vi "Start CANFD Session.vi"(11 "CAN Interface":refnum<k21>="CAN1") -> (0 "Tester Write Session out":refnum<k21>, 1 "Read Session out":refnum<k21>, 3 "DSC Write Session out":refnum<k21>)   [LabVIEW 2018]
uses:
  <vilib>/xnet/xnet.llb/XNET CAN Comm State.ctl
  <vilib>/xnet/xnet.llb/XNET Control Scope.ctl
  <vilib>/xnet/xnet.llb/XNET Frame CAN.ctl
  <vilib>/xnet/xnet.llb/XNET Frame Type CAN.ctl
  <vilib>/xnet/xnet.llb/XNET Create Session (Frame Input Queued).vi
  <vilib>/xnet/xnet.llb/XNET Create Session (Frame Output Single-point).vi
  <vilib>/xnet/xnet.llb/XNET Write (Frame CAN).vi
  <vilib>/xnet/xnet.llb/XNET Read (State CAN Comm).vi
  <vilib>/xnet/xnet.llb/XNET Wait (Interface Communicating).vi
  <resource>/objmgr/xnet.rc
panel:
  in  "error in (no error)":errorcluster
  out "TesterPresentSession":refnum<k21>
  out "CAN:I/O Mode":u32(ring) items=["CAN 2.0", "CAN FD", "CAN FD+BRS"]
  out "Protocol":u32(ring) items=["CAN", "FlexRay", "LIN"]
  out "CAN:Transceiver Capability":u32(ring) items=["HS"=0, "LS"=1, "XS"=3, "XS (HS/LS)"=4]
  out "Interface:CAN:Transceiver State":u32(ring) items=["Normal", "Sleep", "Single Wire Wakeup", "Single Wire High-Speed"]
  out "Interface:CAN:Transceiver State 2":u32(ring) items=["Normal", "Sleep", "Single Wire Wakeup", "Single Wire High-Speed"]
  out "Interface:CAN:Transceiver State 3":u32(ring) items=["Normal", "Sleep", "Single Wire Wakeup", "Single Wire High-Speed"]
  out "CAN:Termination Capability":u32(ring) items=["No", "Yes"]
  out "Array":T1[](array[typedef]) items=["Error Active", "Error Passive", "Bus Off", "Init"]
  out "error out":errorcluster
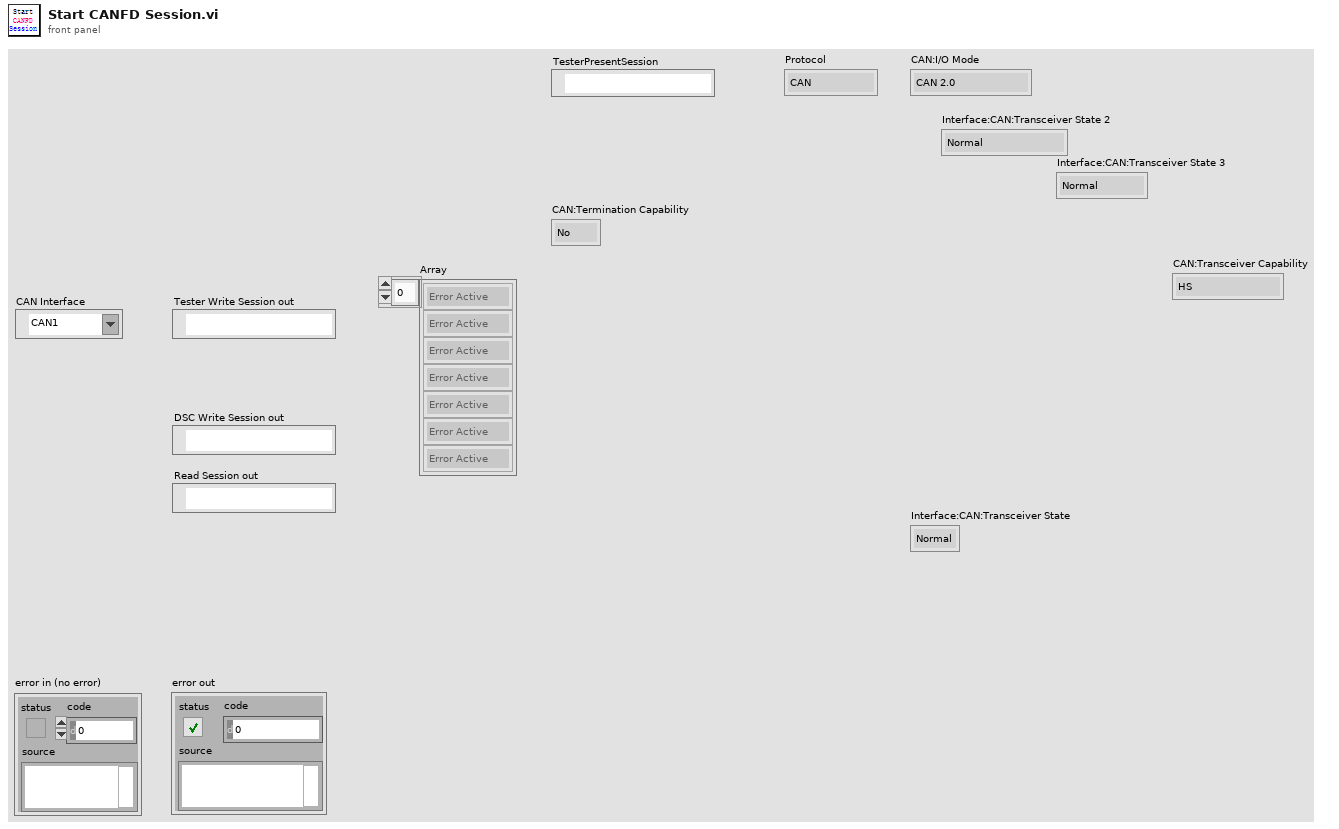
[diagram p1: front panel]
types:
  T1 = typedef "XNET CAN Comm State.ctl" = u8
  T2 = typedef "XNET Frame CAN.ctl" = cluster{"timestamp":timestamp, "payload":u8[], "identifier":u32, "type":T3, "extended?":bool, "echo?":bool}
  T3 = typedef "XNET Frame Type CAN.ctl" = u8
  T4 = typedef "XNET Control Scope.ctl" = u32
  T5 = cluster{"Comment":string, "Default Payload":u8[], "Identifier":u32, "Name (Short)":string, "Payload Length":u32, "PDU_Mapping":cluster{"PDU":string, "Start Bit":u32, "Update Bit":i32}[], "CAN:Extended Identifier?":bool, "CAN:Timing Type":u32, "CAN:Transmit Time":dbl, "CAN:I/O Mode":u32}
  T6 = typedef "XNET CAN Comm.ctl" = cluster{"fault code":i32, "fault?":bool, "communication state":T1, "last error":T7, "receive error counter":u8, "transmit error counter":u8, "transceiver error?":bool, "sleep?":bool}
  T7 = typedef "XNET CAN Last Err.ctl" = u8
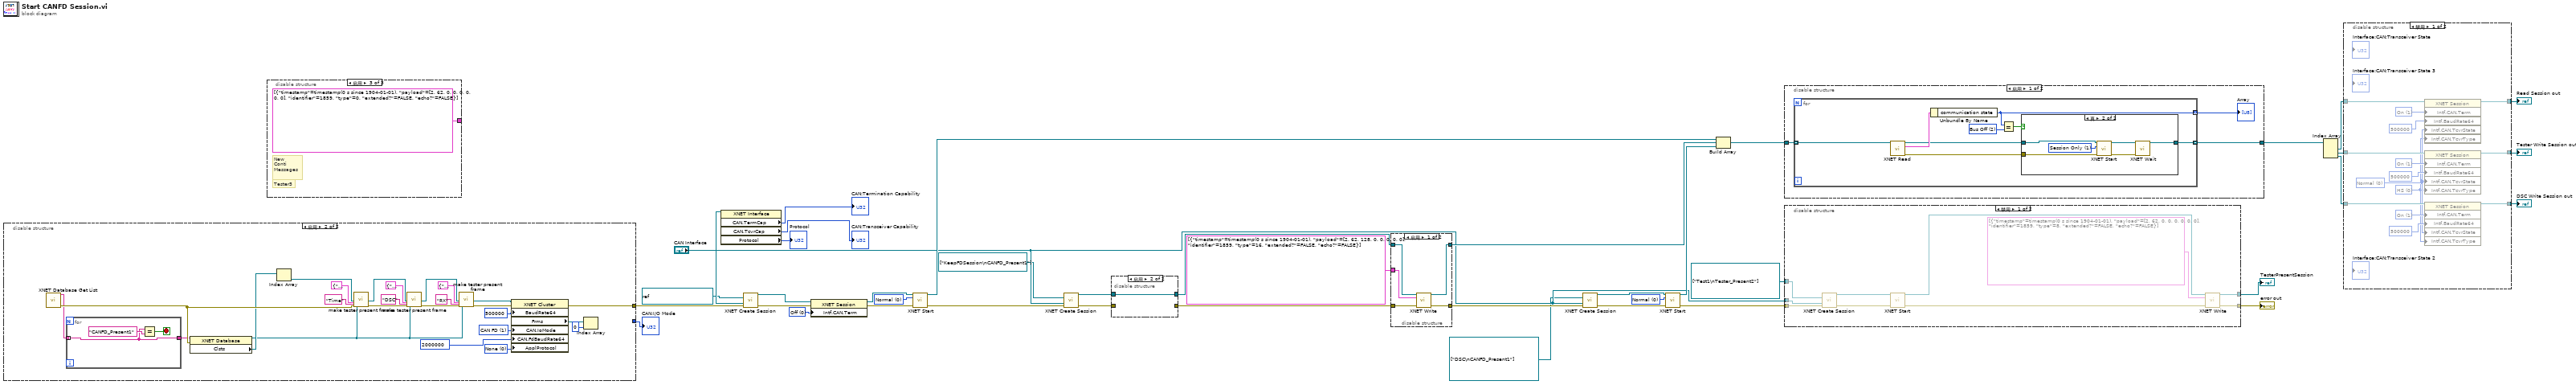
[diagram p0: block diagram]
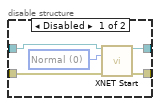
[diagram p3: hidden frame]
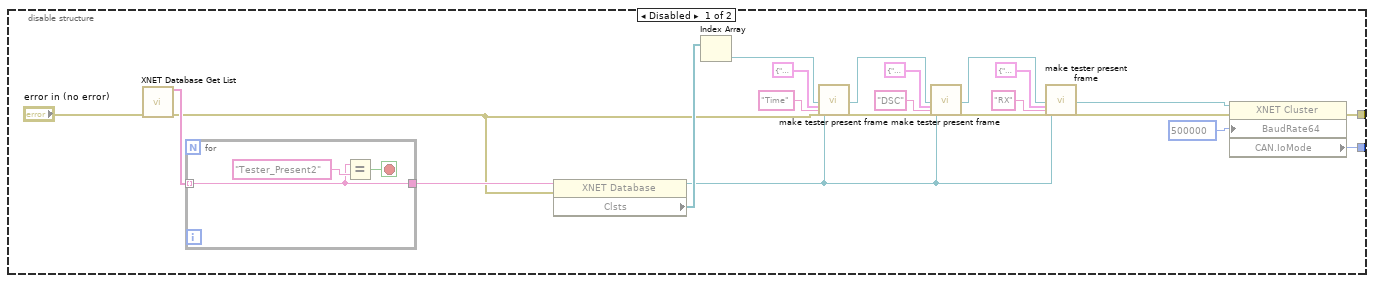
[diagram p4: hidden frame]
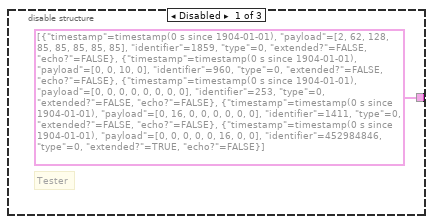
[diagram p9: hidden frame]
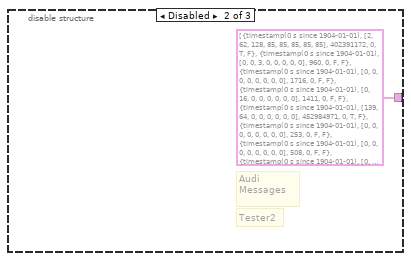
[diagram p10: hidden frame]
diagram:
  w11 = u32 0 items=["Off", "On"] ("Interface:CAN:Termination")
  w29 = T4 0 items=["Normal", "Session Only", "Interface Only", "Session Only Blocking"] ("scope (normal)")
  w30 = T4 0 items=["Normal", "Session Only", "Interface Only", "Session Only Blocking"] ("scope (normal)")
  n1 = disable-structure shown="启用" {
    disable-tunnel: [w60 w69] -> w40
    disable-tunnel: [w41 _] -> w15
    frame Disabled {
      n2 = call <vilib>:"XNET Database Get List.vi"("error in (no error)"="error in (no error)") -> ("array of alias"=w50:string[], "error out"=w46:errorcluster)  [unwired: 12 in, 1 out]
      n3 = for {
        tunnel: w50 -> [w63] mode=indexing
        tunnel: [w63] -> w49
        stop <- w64 stop-if-true
        n4 = Equal?(x=w63, y="Tester_Present2") -> (x = y?=w64:bool)
      }
      n5 = property class="XNET Database"(reference=w49, error in=w46) -> (reference out=w42:refnum<k21>, "Clsts"=w61:refnum<k21>[])  [unwired: 1 out]
      n6 = Index Array(array=w61) -> (element=w44:refnum<k21>)  [unwired: 1 in]
      n7 = call "make tester present frame.vi"("Cluster::"=w44, "New Frame Properties"=T5 {"Comment"="DSC", "Default Payload"=[0, 0, 0, 0, 0, 0, 0, 0], "Identifier"=1714, "Name (Short)"="Time", "Payload Length"=8, "PDU_Mapping"=[], "CAN:Extended Identifier?"=FALSE, "CAN:Timing Type"=0, "CAN:Transmit Time"=0.001, "CAN:I/O Mode"=0}, "frame name"="Time", "error in (no error)"=w46, "database in"=w42) -> ("target cluster out"=w43:refnum<k21>, "error out"=w45:errorcluster)  [unwired: 21 in]
      n8 = call "make tester present frame.vi"("Cluster::"=w43, "New Frame Properties"=T5 {"Comment"="DSC", "Default Payload"=[0, 0, 0, 0, 0, 0, 0, 0], "Identifier"=402391172, "Name (Short)"="DSC", "Payload Length"=8, "PDU_Mapping"=[], "CAN:Extended Identifier?"=TRUE, "CAN:Timing Type"=1, "CAN:Transmit Time"=0.001, "CAN:I/O Mode"=0}, "frame name"="DSC", "error in (no error)"=w45, "database in"=w42) -> ("target cluster out"=w59:refnum<k21>, "error out"=w58:errorcluster)  [unwired: 21 in]
      n9 = call "make tester present frame.vi"("Cluster::"=w59, "New Frame Properties"=T5 {"Comment"="RX", "Default Payload"=[0, 127, 0, 0, 0, 0, 0, 0], "Identifier"=402522244, "Name (Short)"="RX", "Payload Length"=8, "PDU_Mapping"=[], "CAN:Extended Identifier?"=TRUE, "CAN:Timing Type"=1, "CAN:Transmit Time"=0.001, "CAN:I/O Mode"=0}, "frame name"="RX", "error in (no error)"=w58, "database in"=w42) -> ("target cluster out"=w52:refnum<k21>, "error out"=w51:errorcluster)  [unwired: 21 in]
      n10 = property class="XNET Cluster"(reference=w52, error in=w51, "BaudRate64"=u64 500000 ("64bit Baud Rate")) -> (error out=w60:errorcluster, "CAN.IoMode"=w41:u32)  [unwired: 1 out]
    }
    frame Enabled {
      w67 = u32 0 items=["None", "J1939"] ("Application Protocol")
      w68 = u32 1 items=["CAN 2.0", "CAN FD", "CAN FD+BRS"] ("CAN:I/O Mode")
      n11 = call <vilib>:"XNET Database Get List.vi"() -> ("array of alias"=w87:string[], "error out"=w88:errorcluster)  [unwired: 13 in, 1 out]
      n12 = for {
        tunnel: w87 -> [w91] mode=indexing
        tunnel: [w91] -> w74
        stop <- w92 stop-if-true
        n13 = Equal?(x=w91, y="CANFD_Present1") -> (x = y?=w92:bool)
      }
      n14 = property class="XNET Database"(reference=w74, error in=w88) -> (reference out=w71:refnum<k21>, "Clsts"=w75:refnum<k21>[])  [unwired: 1 out]
      n15 = Index Array(array=w75) -> (element=w90:refnum<k21>)  [unwired: 1 in]
      n16 = call "make tester present frame.vi"("Cluster::"=w90, "New Frame Properties"=T5 {"Comment"="Time", "Default Payload"=[0, 0, 0, 0, 0, 0, 0, 0], "Identifier"=1859, "Name (Short)"="Time", "Payload Length"=8, "PDU_Mapping"=[], "CAN:Extended Identifier?"=FALSE, "CAN:Timing Type"=0, "CAN:Transmit Time"=0.1, "CAN:I/O Mode"=0}, "frame name"="Time", "error in (no error)"=w88, "database in"=w71) -> ("target cluster out"=w70:refnum<k21>, "error out"=w89:errorcluster)  [unwired: 21 in]
      n17 = call "make tester present frame.vi"("Cluster::"=w70, "New Frame Properties"=T5 {"Comment"="DSC", "Default Payload"=[0, 0, 0, 16, 1, 0, 0, 0], "Identifier"=1859, "Name (Short)"="DSC", "Payload Length"=8, "PDU_Mapping"=[], "CAN:Extended Identifier?"=FALSE, "CAN:Timing Type"=1, "CAN:Transmit Time"=0.0, "CAN:I/O Mode"=0}, "frame name"="DSC", "error in (no error)"=w89, "database in"=w71) -> ("target cluster out"=w83:refnum<k21>, "error out"=w84:errorcluster)  [unwired: 21 in]
      n18 = call "make tester present frame.vi"("Cluster::"=w83, "New Frame Properties"=T5 {"Comment"="RX", "Default Payload"=[0, 127, 0, 0, 0, 0, 0, 0], "Identifier"=1867, "Name (Short)"="RX", "Payload Length"=8, "PDU_Mapping"=[], "CAN:Extended Identifier?"=FALSE, "CAN:Timing Type"=1, "CAN:Transmit Time"=0.0, "CAN:I/O Mode"=1}, "frame name"="RX", "error in (no error)"=w84, "database in"=w71) -> ("target cluster out"=w85:refnum<k21>, "error out"=w86:errorcluster)  [unwired: 21 in]
      n19 = property class="XNET Cluster"(reference=w85, error in=w86, "BaudRate64"=u64 500000 ("64bit Baud Rate"), "CAN.IoMode"=w68, "CAN.FdBaudRate64"=u64 2000000 ("CAN:64bit FD Baud Rate"), "ApplProtocol"=w67) -> (error out=w69:errorcluster, "Frms"=w73:refnum<k21>[])  [unwired: 1 out]
      n20 = Index Array(array=w73, index=0 ("索引")) -> ()  [unwired: 1 out]
    }
  }
  "CAN:I/O Mode" <- w15
  n21 = disable-structure shown="启用" {
    disable-tunnel: [T2[] [{"timestamp"=timestamp(0 s since 1904-01-01), "payload"=[2, 62, 128, 85, 85, 85, 85, 85], "identifier"=1859, "type"=0, "extended?"=FALSE, "echo?"=FALSE}, {"timestamp"=timestamp(0 s since 1904-01-01), "payload"=[0, 0, 10, 0], "identifier"=960, "type"=0, "extended?"=FALSE, "echo?"=FALSE}, {"timestamp"=timestamp(0 s since 1904-01-01), "payload"=[0, 0, 0, 0, 0, 0, 0, 0], "identifier"=253, "type"=0, "extended?"=FALSE, "echo?"=FALSE}, {"timestamp"=timestamp(0 s since 1904-01-01), "payload"=[0, 16, 0, 0, 0, 0, 0, 0], "identifier"=1411, "type"=0, "extended?"=FALSE, "echo?"=FALSE}, {"timestamp"=timestamp(0 s since 1904-01-01), "payload"=[0, 0, 0, 0, 0, 16, 0, 0], "identifier"=452984846, "type"=0, "extended?"=TRUE, "echo?"=FALSE}] ("data") T2[] [{"timestamp"=timestamp(0 s since 1904-01-01), "payload"=[2, 62, 128, 85, 85, 85, 85, 85], "identifier"=402391172, "type"=0, "extended?"=TRUE, "echo?"=FALSE}, {"timestamp"=timestamp(0 s since 1904-01-01), "payload"=[0, 0, 3, 0, 0, 0, 0, 0], "identifier"=960, "type"=0, "extended?"=FALSE, "echo?"=FALSE}, {"timestamp"=timestamp(0 s since 1904-01-01), "payload"=[0, 0, 0, 0, 0, 0, 0, 0], "identifier"=1716, "type"=0, "extended?"=FALSE, "echo?"=FALSE}, {"timestamp"=timestamp(0 s since 1904-01-01), "payload"=[0, 16, 0, 0, 0, 0, 0, 0], "identifier"=1411, "type"=0, "extended?"=FALSE, "echo?"=FALSE}, {"timestamp"=timestamp(0 s since 1904-01-01), "payload"=[139, 64, 0, 0, 0, 0, 0, 0], "identifier"=452984971, "type"=0, "extended?"=TRUE, "echo?"=FALSE}, {"timestamp"=timestamp(0 s since 1904-01-01), "payload"=[0, 0, 0, 0, 0, 0, 0, 0], "identifier"=253, "type"=0, "extended?"=FALSE, "echo?"=FALSE}, {"timestamp"=timestamp(0 s since 1904-01-01), "payload"=[0, 0, 0, 0, 0, 0, 0, 0], "identifier"=508, "type"=0, "extended?"=FALSE, "echo?"=FALSE}, {"timestamp"=timestamp(0 s since 1904-01-01), "payload"=[0, 0, 0, 0, 150, 0, 0, 0], "identifier"=1646, "type"=0, "extended?"=FALSE, "echo?"=FALSE}, {"timestamp"=timestamp(0 s since 1904-01-01), "payload"=[0, 0, 0, 0, 0, 0, 0, 150], "identifier"=1719, "type"=0, "extended?"=FALSE, "echo?"=FALSE}, {"timestamp"=timestamp(0 s since 1904-01-01), "payload"=[0, 0, 4, 0, 0, 0, 0, 0], "identifier"=958, "type"=0, "extended?"=FALSE, "echo?"=FALSE}, {"timestamp"=timestamp(0 s since 1904-01-01), "payload"=[0, 0, 0, 0, 0, 0, 0, 0], "identifier"=1635, "type"=0, "extended?"=FALSE, "echo?"=FALSE}, {"timestamp"=timestamp(0 s since 1904-01-01), "payload"=[0, 0, 0, 0, 0, 0, 0, 0], "identifier"=319, "type"=0, "extended?"=FALSE, "echo?"=FALSE}, {"timestamp"=timestamp(0 s since 1904-01-01), "payload"=[0, 0, 0, 0, 0, 0, 0, 0], "identifier"=1616, "type"=0, "extended?"=FALSE, "echo?"=FALSE}, {"timestamp"=timestamp(0 s since 1904-01-01), "payload"=[0, 12, 0, 0, 0, 0, 0, 0], "identifier"=1413, "type"=0, "extended?"=FALSE, "echo?"=FALSE}, {"timestamp"=timestamp(0 s since 1904-01-01), "payload"=[0, 0, 0, 0, 0, 0, 0, 0], "identifier"=1462, "type"=0, "extended?"=FALSE, "echo?"=FALSE}, {"timestamp"=timestamp(0 s since 1904-01-01), "payload"=[16, 64, 0, 0, 0, 16, 0, 0], "identifier"=452984848, "type"=0, "extended?"=TRUE, "echo?"=FALSE}, {"timestamp"=timestamp(0 s since 1904-01-01), "payload"=[0, 0, 0, 0, 0, 0, 0, 0], "identifier"=976, "type"=0, "extended?"=FALSE, "echo?"=FALSE}, {"timestamp"=timestamp(0 s since 1904-01-01), "payload"=[0, 0, 0, 0, 0, 0, 0, 0], "identifier"=974, "type"=0, "extended?"=FALSE, "echo?"=FALSE}, {"timestamp"=timestamp(0 s since 1904-01-01), "payload"=[74, 64, 0, 0, 0, 0, 0, 0], "identifier"=452984906, "type"=0, "extended?"=TRUE, "echo?"=FALSE}, {"timestamp"=timestamp(0 s since 1904-01-01), "payload"=[0, 0, 0, 0, 0, 0, 0, 0], "identifier"=977, "type"=0, "extended?"=FALSE, "echo?"=FALSE}, {"timestamp"=timestamp(0 s since 1904-01-01), "payload"=[0, 0, 0, 0, 0, 0, 0, 0], "identifier"=975, "type"=0, "extended?"=FALSE, "echo?"=FALSE}, {"timestamp"=timestamp(0 s since 1904-01-01), "payload"=[75, 64, 0, 0, 0, 0, 0, 0], "identifier"=452984907, "type"=0, "extended?"=TRUE, "echo?"=FALSE}] ("Array 3") T2[] [{"timestamp"=timestamp(0 s since 1904-01-01), "payload"=[2, 62, 0, 0, 0, 0, 0, 0], "identifier"=1859, "type"=0, "extended?"=FALSE, "echo?"=FALSE}] ("data")] -> _
    frame Disabled {
      # "Tester"
    }
    frame Disabled {
      # "Tester2"
      # "Audi\nMessages"
    }
    frame Enabled {
      # "Tester3"
      # "New\nConti\nMessages"
    }
  }
  n22 = property class="XNET Interface"(reference="CAN Interface") -> ("CAN.TermCap"=→"CAN:Termination Capability":u32, "CAN.TcvrCap"=→"CAN:Transceiver Capability":u32, "Protocol"=→"Protocol":u32)  [unwired: 1 in, 2 out]
  n23 = call-poly <vilib>:"XNET Create Session.vi"("frame"=refnum<k21> "RX\nCANFD_Present1" ("XNET Frame"), "interface"="CAN Interface", "error in (no error)"=w40) -> ("session out"=w14:refnum<k21>, "error out"=w12:errorcluster)  [unwired: 11 in]
  n24 = property class="XNET Session"(reference=w14, error in=w12, "Intf.CAN.Term"=w11) -> (reference out=w13:refnum<k21>, error out=w10:errorcluster)
  n25 = call <vilib>:"XNET Start.vi"("session in"=w13, "scope (normal)"=w30, "error in (no error)"=w10) -> ("session out"=w37:refnum<k21>, "error out"=w32:errorcluster)  [unwired: 11 in]
  n26 = call-poly <vilib>:"XNET Create Session.vi"("frame list"=refnum<k21>[] ["KeepFDSession\nCANFD_Present1"] ("Frames"), "interface"="CAN Interface", "error in (no error)"=w32) -> ("session out"=w27:refnum<k21>, "error out"=w28:errorcluster)  [unwired: 11 in]
  n27 = disable-structure shown="启用" {
    disable-tunnel: [w101 w102] -> w39
    disable-tunnel: [w100 _] -> w38
    disable-tunnel: w28 -> [w98 _]
    disable-tunnel: w27 -> [w97 w102]
    frame Disabled {
      w99 = T4 0 items=["Normal", "Session Only", "Interface Only", "Session Only Blocking"] ("scope (normal)")
      n28 = call <vilib>:"XNET Start.vi"("session in"=w97, "scope (normal)"=w99, "error in (no error)"=w98) -> ("session out"=w101:refnum<k21>, "error out"=w100:errorcluster)  [unwired: 11 in]
    }
    frame Enabled {
    }
  }
  n29 = disable-structure shown="启用" {
    disable-tunnel: w39 -> [w107 w108]
    disable-tunnel: w38 -> [w106 w109]
    disable-tunnel: [w105 w108] -> w36
    disable-tunnel: [w104 w109] -> w31
    disable-tunnel: T2[] [{"timestamp"=timestamp(0 s since 1904-01-01), "payload"=[2, 62, 128, 0, 0, 0, 0, 0], "identifier"=1859, "type"=16, "extended?"=FALSE, "echo?"=FALSE}] ("data") -> [w103 _]
    frame Enabled {
      n30 = call-poly <vilib>:"XNET Write.vi"("session in"=w107, "data"=w103, "error in (no error)"=w106) -> ("session out"=w105:refnum<k21>, "error out"=w104:errorcluster)  [unwired: 11 in]
    }
    frame Disabled {
    }
  }
  n31 = call-poly <vilib>:"XNET Create Session.vi"("frame list"=refnum<k21>[] ["DSC\nCANFD_Present1"] ("Frames"), "interface"="CAN Interface", "error in (no error)"=w31) -> ("session out"=w26:refnum<k21>, "error out"=w25:errorcluster)  [unwired: 11 in]
  n32 = call <vilib>:"XNET Start.vi"("session in"=w26, "scope (normal)"=w29, "error in (no error)"=w25) -> ("session out"=w35:refnum<k21>, "error out"=w6:errorcluster)  [unwired: 11 in]
  n33 = Build Array(w37, w36, w35) -> (w34:refnum<k21>[])
  n34 = disable-structure shown="启用" {
    disable-tunnel: w34 -> [w112 w128]
    disable-tunnel: [w110 w128] -> w33
    frame Enabled {
      n35 = for {
        tunnel: w112 -> [w119] mode=indexing
        tunnel: [w114] -> w111 mode=indexing
        tunnel: [w113] -> w110 mode=indexing
        w118 = T1 2 items=["Error Active", "Error Passive", "Bus Off", "Init"] ("y")
        n36 = call-poly <vilib>:"XNET Read.vi"("session in"=w119) -> ("session out"=w116:refnum<k21>, "CAN comm"=w120:T6, "error out"=w115:errorcluster)  [unwired: 12 in]
        n37 = Unbundle By Name(w120) -> ("communication state"=w114:T1)
        n38 = Equal?(x=w114, y=w118) -> (x = y?=w117:bool)
        n39 = case shown="真" w117 {
          tunnel: w116 -> [w121 w127]
          tunnel: w115 -> [_ w125]
          tunnel: [w121 w122] -> w113
          frame False {
          }
          frame True {
            w123 = T4 1 items=["Normal", "Session Only", "Interface Only", "Session Only Blocking"] ("scope (normal)")
            n40 = call <vilib>:"XNET Start.vi"("session in"=w127, "scope (normal)"=w123, "error in (no error)"=w125) -> ("session out"=w126:refnum<k21>, "error out"=w124:errorcluster)  [unwired: 11 in]
            n41 = call-poly <vilib>:"XNET Wait.vi"("session in"=w126, "error in (no error)"=w124) -> ("session out"=w122:refnum<k21>)  [unwired: 12 in, 1 out]
          }
        }
      }
      "Array" <- w111
    }
    frame Disabled {
    }
  }
  n42 = disable-structure shown="禁用" {
    disable-tunnel: "CAN Interface" -> [w138 _]
    disable-tunnel: [w130 _] -> w8
    disable-tunnel: [w131 _] -> w7
    disable-tunnel: refnum<k21>[] ["Test1\nTester_Present2"] ("Frames") -> [w137 _]
    disable-tunnel: w6 -> [w134 _]
    frame Disabled {
      n43 = call-poly <vilib>:"XNET Create Session.vi"("frame list"=w137, "interface"=w138, "error in (no error)"=w134) -> ("session out"=w136:refnum<k21>, "error out"=w135:errorcluster)  [unwired: 11 in]
      n44 = call <vilib>:"XNET Start.vi"("session in"=w136, "error in (no error)"=w135) -> ("session out"=w133:refnum<k21>, "error out"=w132:errorcluster)  [unwired: 12 in]
      n45 = call-poly <vilib>:"XNET Write.vi"("session in"=w133, "data"=T2[] [{"timestamp"=timestamp(0 s since 1904-01-01), "payload"=[2, 62, 0, 0, 0, 0, 0, 0], "identifier"=1859, "type"=8, "extended?"=FALSE, "echo?"=FALSE}], "error in (no error)"=w132) -> ("session out"=w130:refnum<k21>, "error out"=w131:errorcluster)  [unwired: 11 in]
    }
    frame Enabled {
    }
  }
  "error out" <- w7
  "TesterPresentSession" <- w8
  n46 = Index Array(array=w33) -> (element #1=w23:refnum<k21>, element #2=w21:refnum<k21>, element #3=w19:refnum<k21>)  [unwired: 3 in]
  n47 = disable-structure shown="禁用" {
    disable-tunnel: w23 -> [w151 w155]
    disable-tunnel: [w150 w155] -> w22
    disable-tunnel: w21 -> [w147 w154]
    disable-tunnel: [w146 w154] -> w20
    disable-tunnel: w19 -> [w145 w153]
    disable-tunnel: [w144 w153] -> w18
    frame Disabled {
      w139 = u32 0 items=["HS", "LS", "SW", "Ext", "Disc"] ("Interface:CAN:Transceiver Type")
      w140 = u32 0 items=["Normal", "Sleep", "Single Wire Wakeup", "Single Wire High-Speed"] ("Interface:CAN:Transceiver State")
      w148 = u32 1 items=["Off", "On"] ("Interface:CAN:Termination")
      w149 = u32 1 items=["Off", "On"] ("Interface:CAN:Termination")
      w152 = u32 1 items=["Off", "On"] ("Interface:CAN:Termination")
      n48 = property class="XNET Session"(reference=w151, "Intf.CAN.Term"=w152, "Intf.BaudRate64"=u64 500000 ("Interface:64bit Baud Rate"), "Intf.CAN.TcvrState"=w140, "Intf.CAN.TcvrType"=w139) -> (reference out=w150:refnum<k21>)  [unwired: 1 in, 1 out]
      n49 = property class="XNET Session"(reference=w147, "Intf.CAN.Term"=w149, "Intf.BaudRate64"=u64 500000 ("Interface:64bit Baud Rate"), "Intf.CAN.TcvrState"=w140, "Intf.CAN.TcvrType"=w139) -> (reference out=w146:refnum<k21>)  [unwired: 1 in, 1 out]
      n50 = property class="XNET Session"(reference=w145, "Intf.CAN.Term"=w148, "Intf.BaudRate64"=u64 500000 ("Interface:64bit Baud Rate"), "Intf.CAN.TcvrState"=w140, "Intf.CAN.TcvrType"=w139) -> (reference out=w144:refnum<k21>)  [unwired: 1 in, 1 out]
    }
    frame Enabled {
    }
  }
  "Tester Write Session out" <- w20
  "Read Session out" <- w22
  "DSC Write Session out" <- w18
